vi "Halvorsen_ECD_SVI.vi"(0 "Шаг h, с":ext, 1 "n":i32[](array[numeric]), 2 "k":i32, 3 "Parameter_Vector":ext[](array[numeric]), 5 "Время, с":ext, 7 "Initial Conditions":ext[](array[numeric]), 9 "Hmin":ext, 12 "Hmax":ext, 13 "tolerance":ext) -> (4 "Solution":ext[][](array[numeric]))   [LabVIEW 2016]
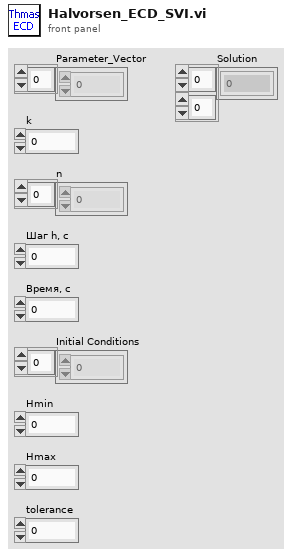
[diagram p1: front panel]
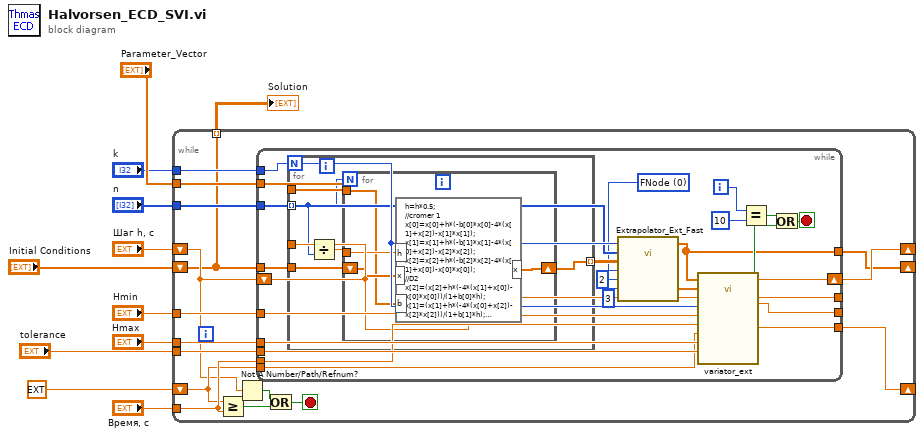
[diagram p0: block diagram]
diagram:
  n1 = while {
    shift-right: [w21] -> _
    shift-left: "Initial Conditions" -> [w12]
    tunnel: "n" -> [w27]
    tunnel: "k" -> [w26]
    shift-right: [w22] -> _
    shift-left: "Шаг h, с" -> [w14]
    shift-right: [w18] -> _
    shift-left: ext 0.0 -> [w19]
    tunnel: "Время, с" -> [w20]
    tunnel: "tolerance" -> [w23]
    tunnel: "Hmin" -> [w25]
    tunnel: "Hmax" -> [w24]
    tunnel: [w12] -> w9 mode=indexing
    tunnel: "Parameter_Vector" -> [w17]
    stop <- w16 stop-if-true
    n2 = Greater Or Equal?(x=w19, y=w20) -> (x >= y?=w15:bool)
    n3 = Not A Number/Path/Refnum?(number/path/refnum=w14) -> (NaN/Path/Refnum?=w13:bool)
    n4 = while {
      tunnel: w25 -> [w44]
      tunnel: w24 -> [w49]
      tunnel: w23 -> [w43]
      tunnel: w26 -> [w47]
      tunnel: w27 -> [w46]
      tunnel: w12 -> [w45]
      shift-right: [w38] -> w22
      shift-left: w14 -> [w30]
      tunnel: [w30] -> _
      tunnel: [w37] -> _
      tunnel: [w36] -> w21
      tunnel: w20 -> [w35]
      tunnel: w19 -> [w34]
      tunnel: [w32] -> w18
      tunnel: w17 -> [w31]
      i -> [w33]
      stop <- w39 stop-if-true
      w28 = u16 0 items=["FNode", "MathScript", "ECD8 Arrays", "ECD8 Fnode", "ECD8 FnodeDiv"] ("Ext.Type")
      n5 = for {
        N: w47 -> [_]
        tunnel: w46 -> [w52] mode=indexing
        tunnel: w30 -> [w57]
        tunnel: w45 -> [w55]
        tunnel: [w56] -> w48 mode=indexing
        tunnel: w31 -> [w53]
        n6 = Divide(x=w57, y=w52) -> (x/y=w54:ext)
        n7 = for {
          N: w52 -> [_]
          shift-right: [w61] -> w56
          shift-left: w55 -> [w60]
          tunnel: w54 -> [w59]
          tunnel: w53 -> [w58]
          n8 = formula code="h=h*0.5;\n//cromer 1\nx[0]=x[0]+h*(-b[0]*x[0]-4*(x[1]+x[2])-x[1]*x[1]);\nx[1]=x[1]+h*(-b[1]*x[1]-4*(x[0]+x[2])-x[2]*x[2]);\nx[2]=x[2]+h*(-b[2]*x[2]-4*(x[1]+x[0])-x[0]*x[0]);\n//D2\nx[2]=(x[2]+h*(-4*(x[1]+x[0])-x[0]*x[0]))/(1+b[0]*h);\nx[1]=(x[1]+h*(-4*(x[0]+x[2])-x[2]*x[2]))/(1+b[1]*h);\nx[0]=(x[0]+h*(-4*(x[1]+x[2])-x[1]*x[1]))/(1+b[2]*h);"("x"=w60, "b"=w58, "h"=w59) -> ("x"=w61:ext[])
        }
      }
      n9 = call "Extrapolator_Ext_Fast.vi"("Порядок экстраполятора"=2 ("Ext. Order"), "Dimension"=3 ("input variable"), "Ext.Type"=w28, "Х - нач. условия"=w48, "n"=w46, "k"=w47) -> ("TPrev"=w50:ext[], "Tout"=w36:ext[])  [unwired: 4 in]
      n10 = call "variator_ext.vi"("Tout"=w36, "tolerance"=w43, "Hmax"=w49, "TPrev"=w50, "Шаг h, с"=w30, "Current time"=w34, "k"=w47, "Hmin"=w44, "tmax"=w35) -> ("Hnew"=w38:ext, "error estimation"=w37:ext, "New time"=w32:ext, "stop"=w40:bool)  [unwired: 3 in]
      n11 = Equal?(x=w33, y=10) -> (x = y?=w41:bool)
      n12 = Or(x=w41, y=w40) -> (x .or. y?=w39:bool)
    }
    n13 = Or(x=w13, y=w15) -> (x .or. y?=w16:bool)
  }
  "Solution" <- w9
